vi "Page - Line.vi"(8 "error in (no error)":errorcluster, 11 "Node Ptr":T2 format="%.0x") -> (0 "error out":errorcluster)   [LabVIEW 2020, in "SLSC-12201 DIO System Explorer.lvlib"]
uses:
  SLSC-12201 DIO System Explorer.lvlib
  <vilib>/NI VeriStand/Custom Device API/Custom Device API.lvlib
  <vilib>/NI VeriStand/Custom Device API/Custom Device Item Ref.ctl
  Direction Control.ctl
panel:
  out "Index":i32
  in  "*Enable":bool
  in  "*Direction":T1 caption="Type" items=["Input", "Output Source", "Output Sink", "Output Push-Pull"]
  in  "SHDocVw.IWebBrowser2":refnum<k7>(container)
  in  "Header":cluster{"Section Name":string}={"Section Name"="Custom Device Item Settings"}
  in  "Description":string
  out "Name":string
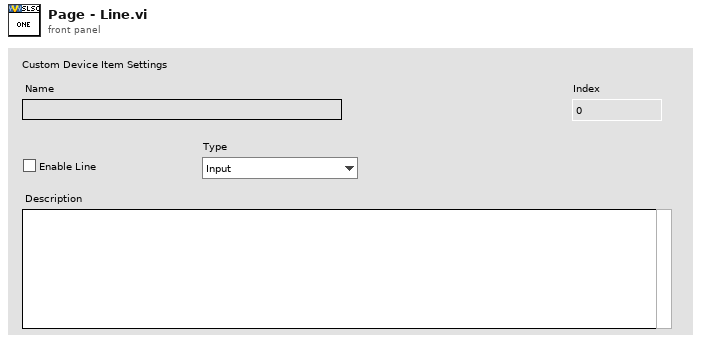
[diagram p1: front panel]
types:
  T1 = typedef "SLSC-12201 DIO System Explorer.lvlib/Direction Control.ctl" = u16
  T2 = typedef "Custom Device API.lvlib/Custom Device Item Ref.ctl" = u64
  T3 = typedef "Custom Device API.lvlib/Custom Device Channel.ctl" = cluster{"Type":T4, "Units":string, "Default Value":dbl, "Faultable":bool, "Scalable":bool}
  T4 = typedef "Custom Device API.lvlib/Custom Device Channel Type.ctl" = enum16{"Input", "Output"}
  T5 = cluster{"Channel Name":string, "SLSC Name":string, "Channel":T3, "Enum Names":string[], "Enum Values":i32[]}[]
  T6 = typedef "Custom Device API.lvlib/Custom Device Item Info.ctl" = cluster{"Name":string, "Is Channel":bool, "GUID":string, "Is Waveform":bool}
  T7 = typedef "Custom Device API.lvlib/Custom Device Commands.ctl" = enum16{"Default", "Item renamed", "Shutdown", "Dynamic button pressed"}
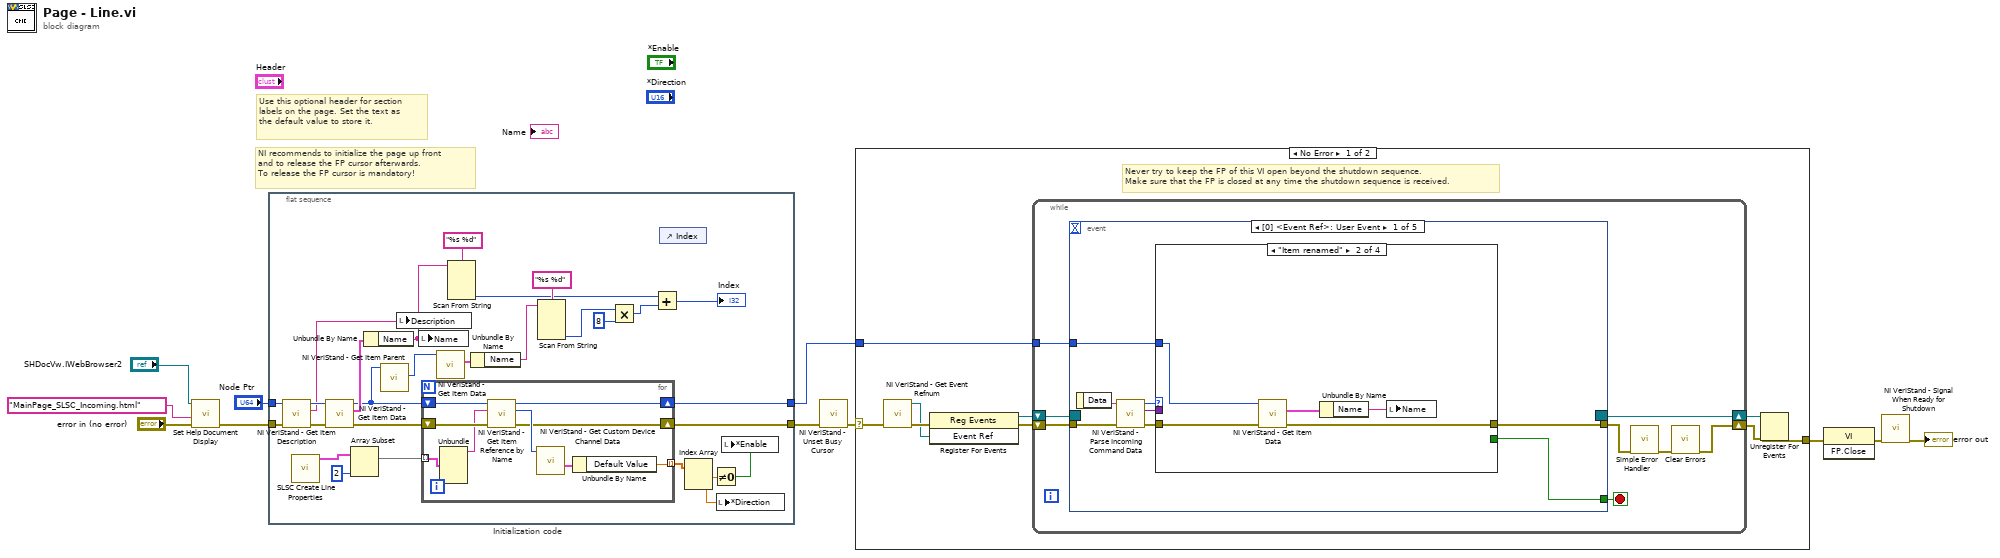
[diagram p0: block diagram]
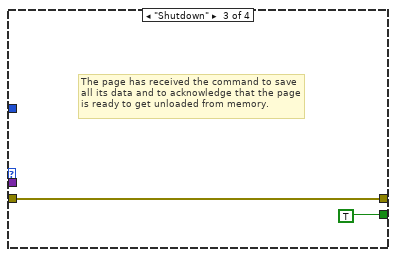
[diagram p3: hidden frame]
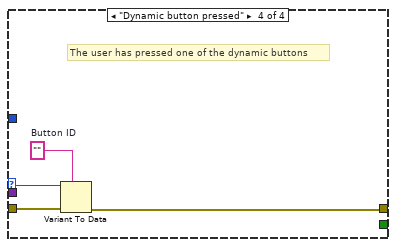
[diagram p4: hidden frame]
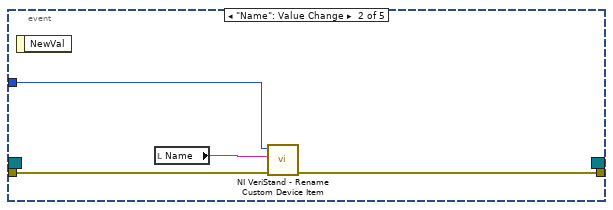
[diagram p5: hidden frame]
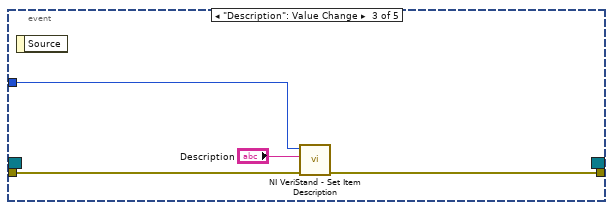
[diagram p6: hidden frame]
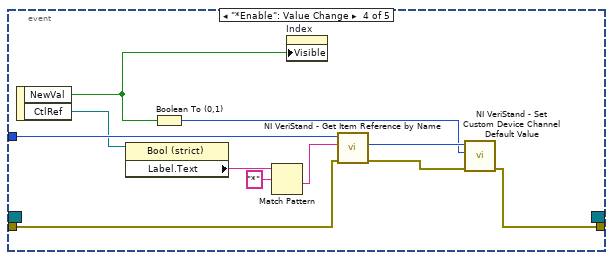
[diagram p7: hidden frame]
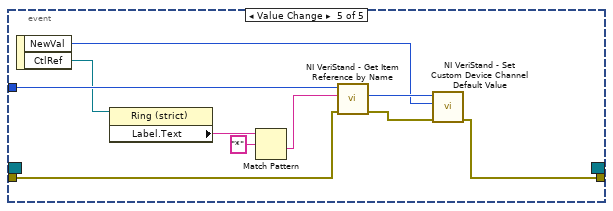
[diagram p8: hidden frame]
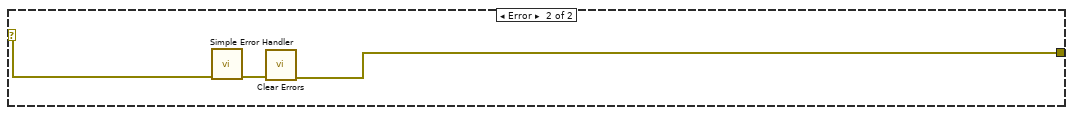
[diagram p9: hidden frame]
diagram:
  # "Use this optional header for section labels on the page. Set the text as the default value to store it."
  # "NI recommends to initialize the page up front\nand to release the FP cursor afterwards.\nTo release the FP cursor is mandatory!"
  n1 = call "Set Help Document Display.vi"("error in (no error)"="error in (no error)", "HTML File to Load"="MainPage_SLSC_Incoming.html" ("HTML File"), "SHDocVw.IWebBrowser2"="SHDocVw.IWebBrowser2") -> ("error out"=w1:errorcluster)  [unwired: 8 in]
  n2 = flat-sequence "Initialization code" {
    tunnel: w1 -> [w38]
    tunnel: "Node Ptr" -> [w37]
    tunnel: [w32] -> w7
    tunnel: [w31] -> w5
    frame #0 {
      n3 = call <vilib>:"NI VeriStand - Get Item Description.vi"("error in (no error)"=w38, "Item Ref in"=w37) -> ("error out"=w35:errorcluster, "Description"=w36:string, "Item Ref out"=w39:T2)  [unwired: 7 out]
      n4 = call "SLSC Create Line Properties.vi"() -> ("Outgoing configuration"=w30:T5)  [unwired: 11 in]
      n5 = call <vilib>:"NI VeriStand - Get Item Data.vi"("error in (no error)"=w35, "Item Ref in"=w39) -> ("error out"=w33:errorcluster, "Item Info"=w34:T6, "Item Ref out"=w25:T2)  [unwired: 7 out]
      n6 = Array Subset(array=w30, length=2) -> (w29:T5)  [unwired: 1 in]
      n7 = Unbundle By Name(w34) -> ("Name"=w26:string)
      n8 = call <vilib>:"NI VeriStand - Get Item Parent.vi"("Item Ref in"=w25) -> ("Parent Ref"=w24:T2)  [unwired: 7 in, 3 out]
      n9 = local write "Description"(w36) -> ()
      n10 = local write "Name"(w26) -> ()
      n11 = for {
        shift-right: [w45] -> w32
        shift-left: w33 -> [w46]
        shift-right: [w43] -> w31
        shift-left: w25 -> [w44]
        tunnel: w29 -> [w42] mode=indexing
        tunnel: [w40] -> w15 mode=indexing
        n12 = Unbundle(w42) -> ("Channel Name"=w41:string)  [unwired: 4 out]
        n13 = call <vilib>:"NI VeriStand - Get Item Reference by Name.vi"("error in (no error)"=w46, "Item Name"=w41, "Parent Ref in"=w44) -> ("error out"=w45:errorcluster, "Item Ref"=w48:T2, "Parent Ref out"=w43:T2)  [unwired: 5 in, 1 out]
        n14 = call <vilib>:"NI VeriStand - Get Custom Device Channel Data.vi"("Channel Ref in"=w48) -> ("Channel"=w47:T3)  [unwired: 5 in, 5 out]
        n15 = Unbundle By Name(w47) -> ("Default Value"=w40:dbl)
      }
      n16 = call <vilib>:"NI VeriStand - Get Item Data.vi"("Item Ref in"=w24) -> ("Item Info"=w23:T6)  [unwired: 1 in, 9 out]
      n17 = Scan From String(format string="%s %d", input string=w26) -> (output 2=w17:i32)  [unwired: 5 in, 3 out]
      n18 = Unbundle By Name(w23) -> ("Name"=w21:string)
      n19 = Scan From String(format string="%s %d", input string=w21) -> (output 2=w20:i32)  [unwired: 5 in, 3 out]
      n20 = Multiply(x=w20, y=8) -> (x*y=w18:i32)
      n21 = Add(x=w17, y=w18) -> (x+y=→"Index":i32)
      n22 = control-ref of="Index"() -> ()  [unwired: 1 out]
      n23 = Index Array(array=w15) -> (element #1=w14:dbl, element #2=w12:dbl)  [unwired: 2 in]
      n24 = Not Equal To 0?(x=w14) -> (x != 0?=w13:bool)
      n25 = local write "*Direction"(w12) -> ()
      n26 = local write "*Enable"(w13) -> ()
    }
  }
  n27 = call <vilib>:"NI VeriStand - Unset Busy Cursor.vi"("error in (no error)"=w7) -> ("error out"=w6:errorcluster)  [unwired: 10 out]
  n28 = case shown="No Error" w6 {
    selector: w6 -> [w49 w117]
    tunnel: [w54 w115] -> w11
    tunnel: w5 -> [w50 _]
    frame No Error {
      # "Never try to keep the FP of this VI open beyond the shutdown sequence.\nMake sure that the FP is closed at any time the shutdown sequence is received."
      n29 = call <vilib>:"NI VeriStand - Get Event Refnum.vi"("error in (no error)"=w49) -> ("error out"=w57:errorcluster, "Event Ref"=w53:refnum<user-event>)  [unwired: 9 out]
      n30 = register-events(error in=w57, w53) -> (reference out=w51:refnum<event-registration>, error out=w52:errorcluster)  [unwired: 1 in]
      n31 = while {
        tunnel: w50 -> [w61]
        shift-right: [w58] -> w55
        shift-left: w52 -> [w64]
        shift-right: [w65] -> w56
        shift-left: w51 -> [w63]
        stop <- w62 stop-if-true
        n32 = event shown="[0] <Event Ref>: User Event" {
          selector: w63 -> [_ _ _ _ _]
          dyn-events: [_ _ _ _ _] -> w65
          timeout: _ -> [_ _ _ _ _]
          tunnel: w64 -> [w73 w89 w92 w101 w112]
          tunnel: [w69 _ _ _ _] -> w62
          tunnel: [w68 w88 w91 w99 w110] -> w60
          tunnel: w61 -> [w67 w87 w93 w104 w114]
          event User Event {
            n33 = event-data() -> ("Data"=w72:string)  [unwired: 1 out]
            n34 = call <vilib>:"NI VeriStand - Parse Incoming Command Data.vi"("error in (no error)"=w73, "Incoming data"=w72) -> ("error out"=w71:errorcluster, "Outgoing data"=w66:variant, "Action"=w70:T7)  [unwired: 7 out]
            n35 = case shown="\"Item renamed\"" w70 {
              tunnel: w71 -> [w74 w79 w80 w85]
              tunnel: [_ _ TRUE _] -> w69
              tunnel: [w74 w76 w80 w82] -> w68
              tunnel: w67 -> [_ w78 _ _]
              tunnel: w66 -> [_ _ _ w84]
              frame "Default", Default {
              }
              frame "Item renamed" {
                n36 = call <vilib>:"NI VeriStand - Get Item Data.vi"("error in (no error)"=w79, "Item Ref in"=w78) -> ("error out"=w76:errorcluster, "Item Info"=w77:T6)  [unwired: 8 out]
                n37 = Unbundle By Name(w77) -> ("Name"=w75:string)
                n38 = local write "Name"(w75) -> ()
              }
              frame "Shutdown" {
                # "The page has received the command to save all its data and to acknowledge that the page is ready to get unloaded from memory."
              }
              frame "Dynamic button pressed" {
                w83 = ""  # Button ID
                # "The user has pressed one of the dynamic buttons"
                n39 = Variant To Data(error in=w85, type=w83, Variant=w84) -> (error out=w82:errorcluster)  [unwired: 1 out]
              }
            }
          }
          event "Name": Value Change {
            n40 = event-data() -> ()  [unwired: 2 out]
            n41 = local read "Name"() -> (w86:string)
            n42 = call <vilib>:"NI VeriStand - Rename Custom Device Item.vi"("error in (no error)"=w89, "New Name"=w86, "Item Ref in"=w87) -> ("error out"=w88:errorcluster)  [unwired: 1 in, 7 out]
          }
          event "Description": Value Change {
            n43 = event-data() -> ()  [unwired: 2 out]
            n44 = call <vilib>:"NI VeriStand - Set Item Description.vi"("error in (no error)"=w92, "Description"="Description", "Item Ref in"=w93) -> ("error out"=w91:errorcluster)  [unwired: 8 out]
          }
          event "*Enable": Value Change {
            n45 = event-data() -> ("NewVal"=w94:bool, "CtlRef"=w96:refnum<vi>)  [unwired: 1 out]
            n46 = property class="Bool (strict)"(reference=w96) -> ("Label.Text"=w98:string)  [unwired: 1 in, 2 out]
            n47 = Boolean To (0,1)(Boolean=w94) -> (0, 1=w102:i16)
            n48 = Match Pattern(string=w98, regular expression="*") -> (after substring=w95:string)  [unwired: 1 in, 3 out]
            n49 = property on="Index" class="DigNum (strict)"("Visible"=w94) -> ()  [unwired: 2 in, 2 out]
            n50 = call <vilib>:"NI VeriStand - Get Item Reference by Name.vi"("error in (no error)"=w101, "Item Name"=w95, "Parent Ref in"=w104) -> ("error out"=w100:errorcluster, "Item Ref"=w103:T2)  [unwired: 5 in, 2 out]
            n51 = call <vilib>:"NI VeriStand - Set Custom Device Channel Default Value.vi"("error in (no error)"=w100, "Default Value"=w102, "Channel Ref in"=w103) -> ("error out"=w99:errorcluster)  [unwired: 7 in, 1 out]
          }
          event Value Change {
            n52 = event-data() -> ("NewVal"=w105:T1, "CtlRef"=w109:refnum<vi>)  [unwired: 1 out]
            n53 = property class="Ring (strict)"(reference=w109) -> ("Label.Text"=w108:string)  [unwired: 1 in, 2 out]
            n54 = Match Pattern(string=w108, regular expression="*") -> (after substring=w106:string)  [unwired: 1 in, 3 out]
            n55 = call <vilib>:"NI VeriStand - Get Item Reference by Name.vi"("error in (no error)"=w112, "Item Name"=w106, "Parent Ref in"=w114) -> ("error out"=w111:errorcluster, "Item Ref"=w113:T2)  [unwired: 5 in, 2 out]
            n56 = call <vilib>:"NI VeriStand - Set Custom Device Channel Default Value.vi"("error in (no error)"=w111, "Default Value"=w105, "Channel Ref in"=w113) -> ("error out"=w110:errorcluster)  [unwired: 7 in, 1 out]
          }
        }
        n57 = call <vilib>:"Simple Error Handler.vi"("error in (no error)"=w60) -> ("error out"=w59:errorcluster)  [unwired: 1 in, 7 out]
        n58 = call <vilib>:"Clear Errors.vi"("error in (no error)"=w59) -> ("error out"=w58:errorcluster)  [unwired: 1 in, 5 out]
      }
      n59 = Unregister For Events(event registration refnum=w56, error in=w55) -> (error out=w54:errorcluster)
    }
    frame Error {
      n60 = call <vilib>:"Simple Error Handler.vi"("error in (no error)"=w117) -> ("error out"=w116:errorcluster)  [unwired: 1 in, 7 out]
      n61 = call <vilib>:"Clear Errors.vi"("error in (no error)"=w116) -> ("error out"=w115:errorcluster)  [unwired: 1 in, 5 out]
    }
  }
  n62 = invoke class="VI" method="FP.Close"(error in=w11) -> (error out=w10:errorcluster)  [unwired: 2 in, 2 out]
  n63 = call <vilib>:"NI VeriStand - Signal When Ready for Shutdown.vi"("error in (no error)"=w10) -> ("error out"=→"error out":errorcluster)  [unwired: 10 out]
